vi "Stop simulation.vi"() -> ()   [LabVIEW 2019]
panel:
  in  "Boolean 3":bool
  out "Boolean 2":bool
  out "Boolean":bool
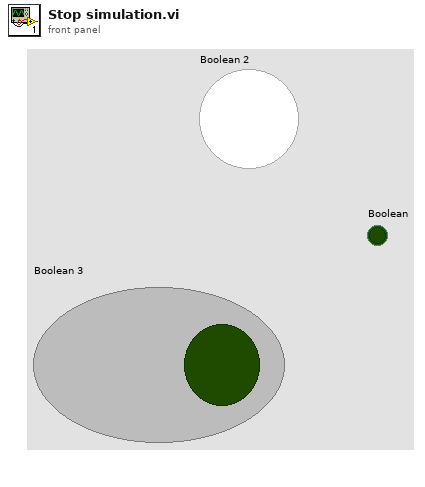
[diagram p1: front panel]
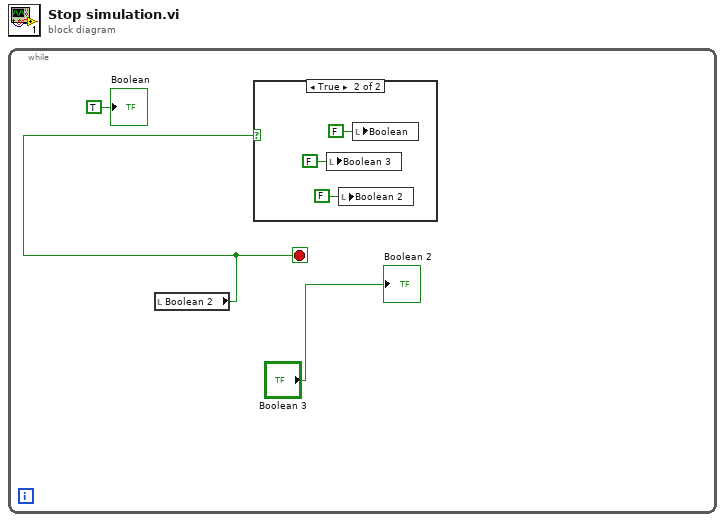
[diagram p0: block diagram]
diagram:
  n1 = while {
    stop <- w1 stop-if-true
    n2 = local read "Boolean 2"() -> (w1:bool)
    n3 = case shown="True" w1 {
      frame False {
      }
      frame True {
        n4 = local write "Boolean 3"(FALSE ("Boolean 2")) -> ()
        n5 = local write "Boolean 2"(FALSE ("Boolean 2")) -> ()
        n6 = local write "Boolean"(FALSE ("Boolean")) -> ()
      }
    }
    "Boolean" <- TRUE ("Boolean")
    "Boolean 2" <- "Boolean 3"
  }
